vi "Send Synced Scrolls.vi"(8 "error in (no error)":errorcluster, 11 "2DArrayManager in":refnum<class "2DArrayManager.lvclass">) -> (0 "error out":errorcluster, 3 "2DArrayManager out":refnum<class "2DArrayManager.lvclass">, 4 "Sync Response":refnum<notifier>)   [LabVIEW 2020, in "OOPanel.lvlib" / "2DArrayManager.lvclass"]
uses:
  2DArrayManager.lvclass
  2DArrayManager.lvclass/2DArrayManager.ctl
  Synced Scroll.ctl
  2D Position.ctl
  Direction.ctl
  OOPanel.lvlib
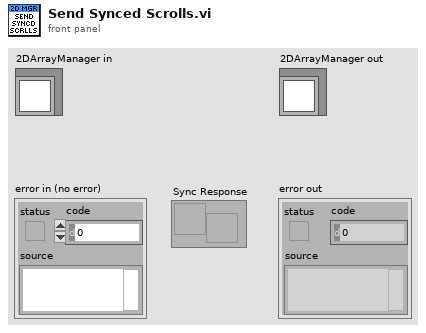
[diagram p1: front panel]
types:
  T1 = typedef "OOPanel.lvlib/2DArrayManager.lvclass/State.ctl" = cluster{"Scroll":T2, "Scroll Max":T2, "Top-Left Index":T3, "H Scroll Sync":refnum<user-event>, "V Scroll Sync":refnum<user-event>, "Sync":bool, "H Scroll Vis":bool, "V Scroll Vis":bool, "Blank Pool":refnum<queue>}
  T2 = typedef "OOPanel.lvlib/2D Position.ctl" = cluster{"H":i32, "V":i32}
  T3 = typedef "OOPanel.lvlib/2D Index.ctl" = cluster{"Row":i32, "Col":i32}
  T4 = typedef "OOPanel.lvlib/2DArrayManager.lvclass/Synced Scroll.ctl" = cluster{"Position":T2, "Direction":T5, "Sync Response":refnum<notifier>}
  T5 = typedef "OOPanel.lvlib/Direction.ctl" = enum16{"Vertical", "Horizontal", "Both"}
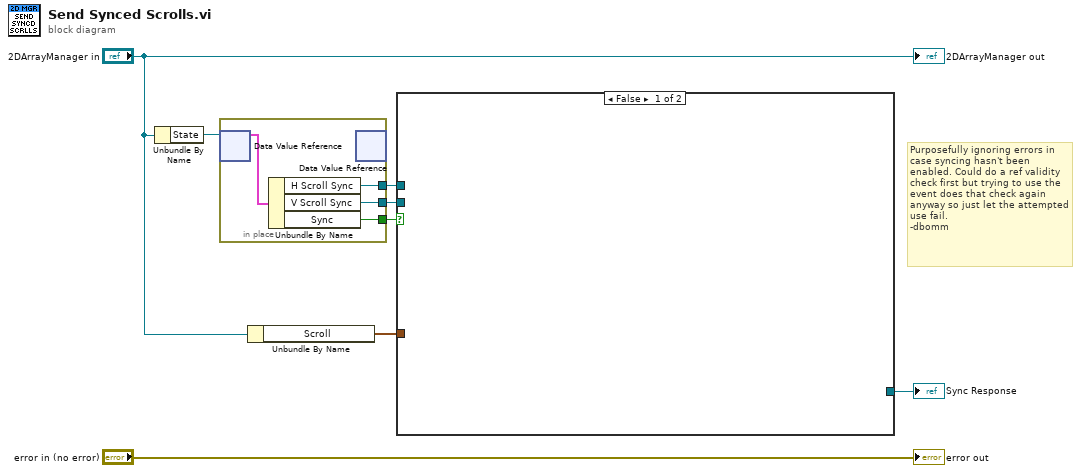
[diagram p0: block diagram]
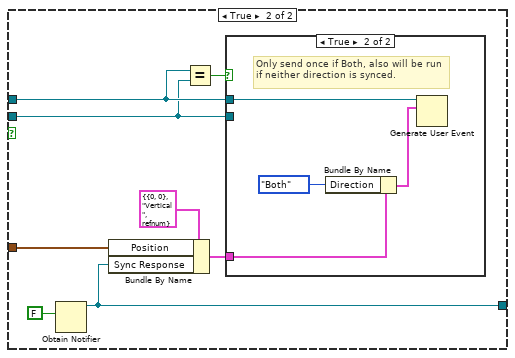
[diagram p2: hidden frame]
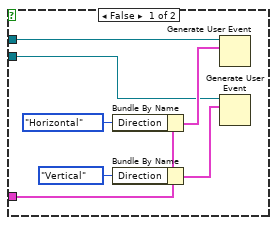
[diagram p3: hidden frame]
diagram:
  # "Purposefully ignoring errors in case syncing hasn't been enabled. Could do a ref validity check first but trying to use the event does that check again anyway so just let the attempted use fail.\n-dbomm"
  n1 = Unbundle By Name("2DArrayManager in") -> ("State"=w7:refnum<data-value>)
  n2 = in-place {
    in-place-border: [w11] -> w4
    in-place-border: [w10] -> w3
    in-place-border: [w9] -> w1
    n3 = in-place-dvr #1(w7) -> (w12:T1)  [unwired: 1 out]
    n4 = Unbundle By Name(w12) -> ("H Scroll Sync"=w11:refnum<user-event>, "V Scroll Sync"=w10:refnum<user-event>, "Sync"=w9:bool)
    n5 = in-place-dvr #1() -> ()  [unwired: 1 in, 2 out]
  }
  n6 = Unbundle By Name("2DArrayManager in") -> ("Scroll"=w5:T2)
  n7 = case shown="False" w1 {
    tunnel: w5 -> [_ w19]
    tunnel: w4 -> [_ w16]
    tunnel: w3 -> [_ w15]
    tunnel: [_ w13] -> w2
    frame False {
    }
    frame True {
      n8 = Obtain Notifier(notification data type=FALSE) -> (notifier out=w13:refnum<notifier>)  [unwired: 3 in, 2 out]
      n9 = Bundle By Name(cluster=T4 {"Position"={"H"=0, "V"=0}, "Direction"=enum."Vertical", "Sync Response"=refnum} ("Synced Scroll"), "Position"=w19, "Sync Response"=w13) -> (w17:T4)
      n10 = Equal?(x=w16, y=w15) -> (x = y?=w18:bool)
      n11 = case shown="True" w18 {
        tunnel: w17 -> [w25 w31]
        tunnel: w16 -> [w24 w29]
        tunnel: w15 -> [w22 _]
        frame False {
          n12 = Bundle By Name(cluster=w25, "Direction"=Direction."Horizontal") -> (w23:T4)
          n13 = Bundle By Name(cluster=w25, "Direction"=Direction."Vertical") -> (w21:T4)
          n14 = Generate User Event(user event=w24, event data cluster=w23) -> ()  [unwired: 2 in, 2 out]
          n15 = Generate User Event(user event=w22, event data cluster=w21) -> ()  [unwired: 2 in, 2 out]
        }
        frame True {
          # "Only send once if Both, also will be run if neither direction is synced."
          n16 = Bundle By Name(cluster=w31, "Direction"=Direction."Both") -> (w28:T4)
          n17 = Generate User Event(user event=w29, event data cluster=w28) -> ()  [unwired: 2 in, 2 out]
        }
      }
    }
  }
  "Sync Response" <- w2
  "error out" <- "error in (no error)"
  "2DArrayManager out" <- "2DArrayManager in"
